vi "Create Annotation File Name.vi"(11 "Subject Number":string) -> (3 "File Name":string)   [LabVIEW 2021]
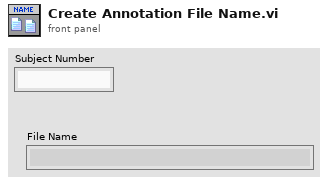
[diagram p1: front panel]
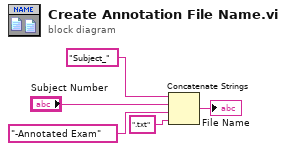
[diagram p0: block diagram]
diagram:
  n1 = Concatenate Strings("Subject_" ("string"), "Subject Number", "-Annotated Exam" ("string"), ".txt" ("string")) -> (→"File Name":string)
